vi "LightFieldAcquireBackground.vi"(5 "Cycle time\n(ms)":i32=3 min=0 step=1, 6 "File Exists":bool, 7 "On CCD Acc.":i32=3 min=0 step=1, 8 "error in":errorcluster, 9 "BIN":u16(ring)=2 items=["1x1", "2x2", "4x4"], 10 "MODE":u16(ring) items=["Normal", "DIF"], 11 "VISA resource name":refnum<visa-resource-name>) -> (0 "error out":errorcluster, 3 "VISA resource name out":refnum<visa-resource-name>)   [LabVIEW 2018]
uses:
  user32.dll
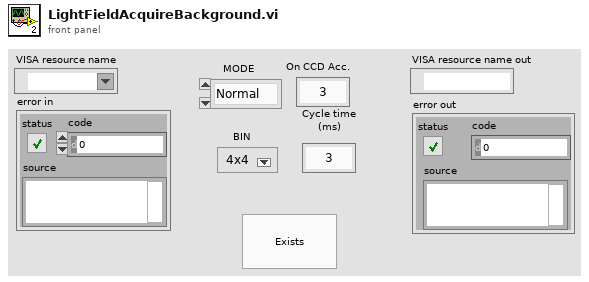
[diagram p1: front panel]
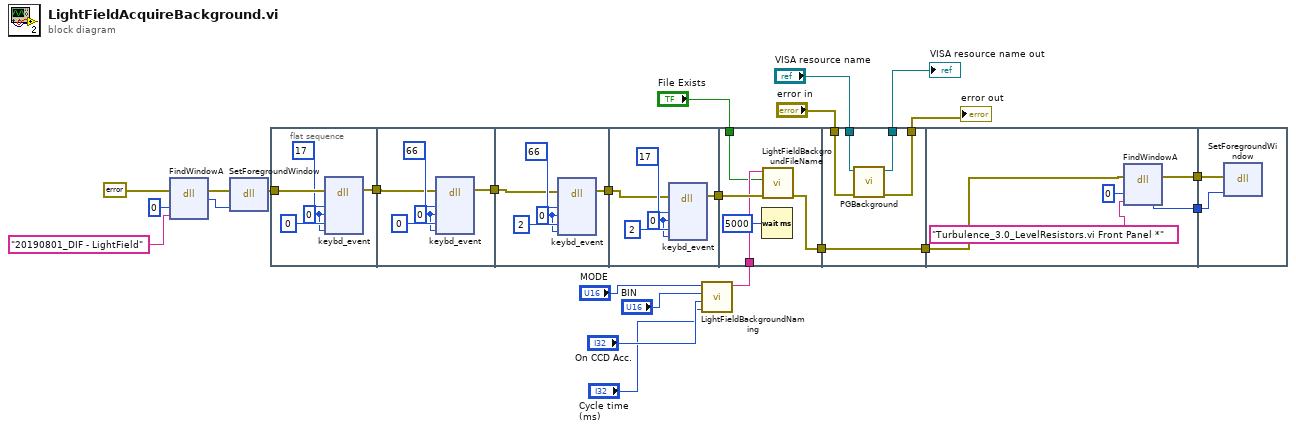
[diagram p0: block diagram]
diagram:
  n1 = dll-call lib="user32.dll" fn="FindWindowA"(error in=errorcluster {"status"=FALSE, "code"=0, "source"=""} ("error in (no error)"), "IpszClassName"=0, "IpszWindowName"="20190801_DIF - LightField") -> (error out=w24:errorcluster, "hWnd"=w23:u32)  [unwired: 4 in, 1 out]
  n2 = dll-call lib="user32.dll" fn="SetForegroundWindow"(error in=w24, "Handle"=w23) -> (error out=w19:errorcluster)  [unwired: 4 in, 1 out]
  n3 = flat-sequence {
    tunnel: w19 -> [w29]
    tunnel: [w25] -> w16
    tunnel: w16 -> [w31]
    tunnel: [w30] -> w17
    tunnel: w17 -> [w36]
    tunnel: [w35] -> w18
    tunnel: w18 -> [w41]
    tunnel: [w40] -> w15
    tunnel: w15 -> [w49]
    tunnel: w6 -> [w48]
    tunnel: [w47] -> w14
    tunnel: "File Exists" -> [w45]
    tunnel: w14 -> [w54]
    tunnel: "error in" -> [w53]
    tunnel: "VISA resource name" -> [w52]
    tunnel: [w51] -> w11
    tunnel: [w50] -> w10
    tunnel: [w54] -> w9
    tunnel: w9 -> [w55]
    tunnel: [w57] -> w8
    tunnel: [w56] -> w7
    tunnel: w8 -> [w60]
    tunnel: w7 -> [w61]
    frame #0 {
      w26 = u8 0 ("bScan")
      n4 = dll-call lib="user32.dll" fn="keybd_event"(error in=w29, "bVk"=17, "bScan"=w26, "dwFlags"=0, "dwExtraInfo"=w26) -> (error out=w25:errorcluster)  [unwired: 7 in, 1 out]
    }
    frame #1 {
      w32 = u8 0 ("bScan")
      n5 = dll-call lib="user32.dll" fn="keybd_event"(error in=w31, "bVk"=66, "bScan"=w32, "dwFlags"=0, "dwExtraInfo"=w32) -> (error out=w30:errorcluster)  [unwired: 7 in, 1 out]
    }
    frame #2 {
      w37 = u8 0 ("bScan")
      n6 = dll-call lib="user32.dll" fn="keybd_event"(error in=w36, "bVk"=66, "bScan"=w37, "dwFlags"=2, "dwExtraInfo"=w37) -> (error out=w35:errorcluster)  [unwired: 7 in, 1 out]
    }
    frame #3 {
      w42 = u8 0 ("bScan")
      n7 = dll-call lib="user32.dll" fn="keybd_event"(error in=w41, "bVk"=17, "bScan"=w42, "dwFlags"=2, "dwExtraInfo"=w42) -> (error out=w40:errorcluster)  [unwired: 7 in, 1 out]
    }
    frame #4 {
      n8 = Wait (ms)(milliseconds to wait=u32 5000) -> ()  [unwired: 1 out]
      n9 = call "LightFieldBackgroundFileName.vi"("error in"=w49, "File Exists"=w45, "FileName"=w48) -> ("error out"=w47:errorcluster)  [unwired: 8 in]
    }
    frame #5 {
      n10 = call "PGBackground.vi"("error in"=w53, "VISA resource name"=w52) -> ("error out"=w50:errorcluster, "VISA resource name out"=w51:refnum<visa-resource-name>)  [unwired: 8 in]
    }
    frame #6 {
      n11 = dll-call lib="user32.dll" fn="FindWindowA"(error in=w55, "IpszClassName"=0, "IpszWindowName"="Turbulence_3.0_LevelResistors.vi Front Panel *") -> (error out=w57:errorcluster, "hWnd"=w56:u32)  [unwired: 4 in, 1 out]
    }
    frame #7 {
      n12 = dll-call lib="user32.dll" fn="SetForegroundWindow"(error in=w60, "Handle"=w61) -> ()  [unwired: 4 in, 2 out]
    }
  }
  n13 = call "LightFieldBackgroundNaming.vi"("Cycle time\n(ms)"="Cycle time\n(ms)", "On CCD Acc."="On CCD Acc.", "BIN"="BIN", "MODE"="MODE") -> ("Background File Name"=w6:string)  [unwired: 5 in, 2 out]
  "VISA resource name out" <- w11
  "error out" <- w10
